vi "Logitech Camera.vi"() -> ()   [LabVIEW 2012]
uses:
  <vilib>/Utility/sysdir.llb/System Directory Type.ctl
panel:
  in  "error in":errorcluster
  out "error out":errorcluster
  out "Lines":T1(array[cluster]) {"End Point"."Y" format="%.2f"; "End Point"."X" format="%.2f"; "Start Point"."Y" format="%.2f"; "Start Point"."X" format="%.2f"}
  in  "stop?":bool caption="Stop (F)"
  out "Image Out":T2(plugin-control)
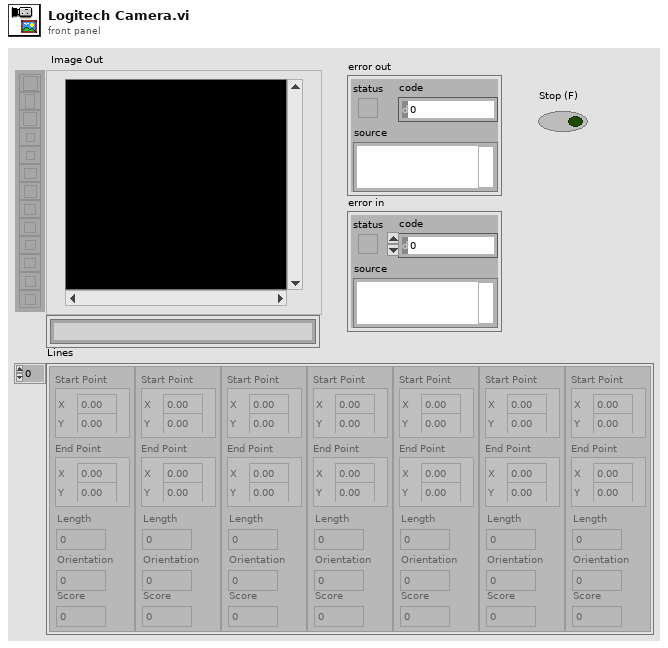
[diagram p1: front panel]
types:
  T1 = cluster{"Start Point":cluster{"X":sgl, "Y":sgl}, "End Point":cluster{"X":sgl, "Y":sgl}, "Length":dbl, "Orientation":dbl, "Score":dbl}[]
  T2 = typedef "IMAQ Image.ctl" = refnum<image>
  T3 = typedef "System Directory Type.ctl" = i32
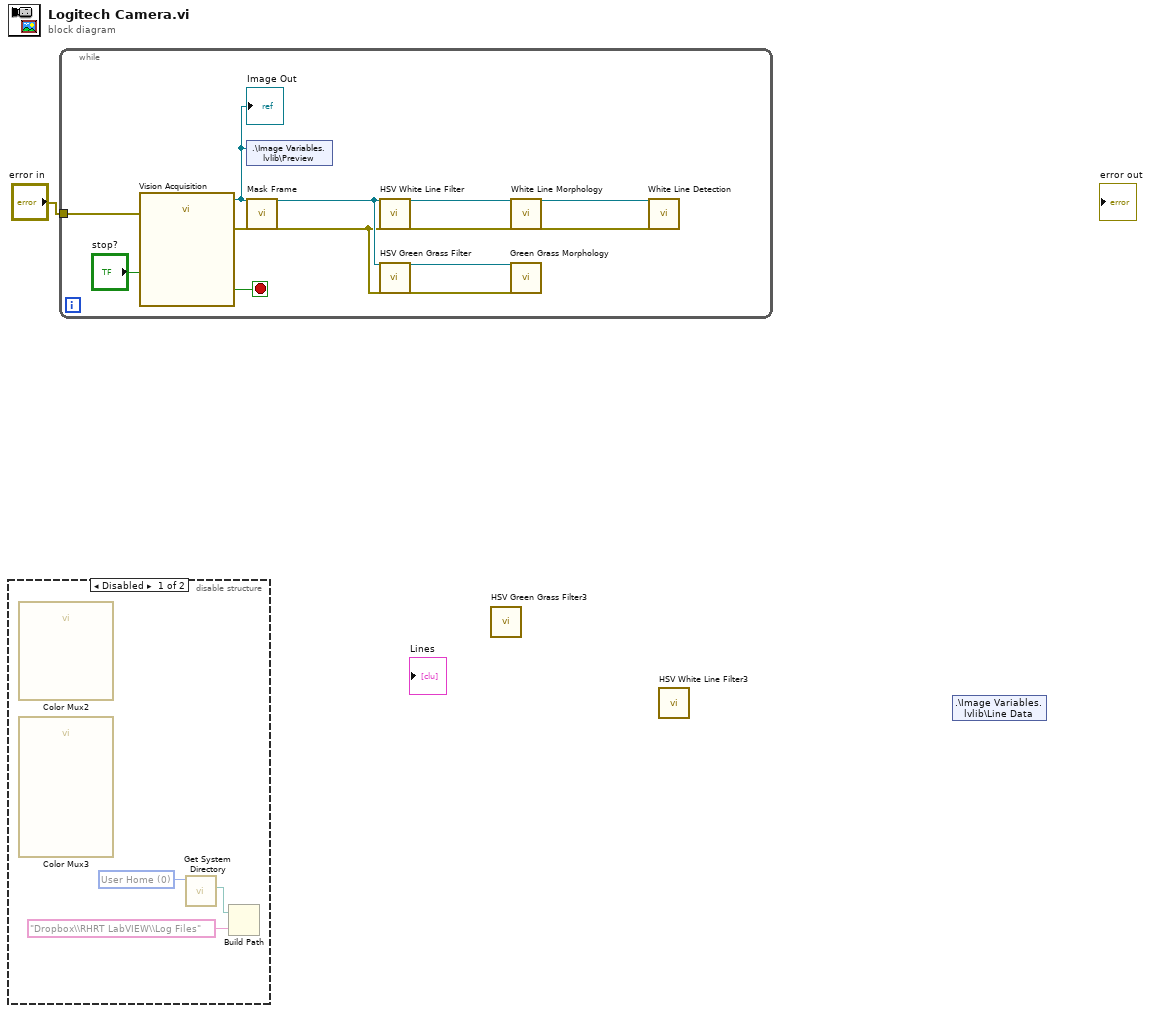
[diagram p0: block diagram]
diagram:
  n1 = disable-structure shown="Disabled" {
    frame Disabled {
      w2 = T3 0 items=["User Home"=0, "User Desktop"=1, "User Documents"=2, "User Application Data"=3, "User Preferences"=4, "User Temporary"=5, "Public Documents"=6, "Public Application Data"=7, "Public Preferences"=8, "Public Cache"=13, "System Core Libraries"=9, "System Installed Libraries"=10, "Application Files"=11, "Boot Volume Root"=12] ("system directory type")
      n2 = call "Color Mux2"() -> ()  [unwired: 26 in, 2 out]
      n3 = call "Color Mux3"() -> ()  [unwired: 23 in, 5 out]
      n4 = call <vilib>:"Get System Directory.vi"("system directory type"=w2) -> ("system directory"=w3:path)  [unwired: 10 in]
      n5 = Build Path(base path=w3, name or relative path="Dropbox\\RHRT LabVIEW\\Log Files") -> ()  [unwired: 1 out]
    }
    frame Enabled {
    }
  }
  n6 = while {
    tunnel: "error in" -> [w15]
    stop <- w16 stop-if-true
    n7 = call "Vision Acquisition"("Stop (F)"="stop?", "error in"=w15) -> ("Image Out"=w14:T2, "Stopped"=w16:bool, "error out"=w13:errorcluster)  [unwired: 23 in]
    "Image Out" <- w14
    n8 = shared-variable ".\\Image Variables.lvlib\\Preview"(w14) -> ()  [unwired: 1 in, 1 out]
    n9 = call "Mask Frame"("Image In"=w14, "error in"=w13) -> ("Image Out"=w8:T2, "error out"=w7:errorcluster)  [unwired: 24 in]
    n10 = call "HSV White Line Filter"("Image In"=w8, "error in"=w7) -> ("Image Out"=w12:T2, "error out"=w11:errorcluster)  [unwired: 24 in]
    n11 = call "HSV Green Grass Filter"("Image In"=w8, "error in"=w7) -> ("Image Out"=w6:T2, "error out"=w5:errorcluster)  [unwired: 24 in]
    n12 = call "White Line Morphology"("Image In"=w12, "error in"=w11) -> ("Image Out"=w10:T2, "error out"=w9:errorcluster)  [unwired: 24 in]
    n13 = call "Green Grass Morphology"("Image In"=w6, "error in"=w5) -> ()  [unwired: 24 in, 2 out]
    n14 = call "White Line Detection"("Image In"=w10, "error in"=w9) -> ()  [unwired: 22 in, 4 out]
  }
  n15 = call "HSV Green Grass Filter3"() -> ()  [unwired: 26 in, 2 out]
  n16 = call "HSV White Line Filter3"() -> ()  [unwired: 24 in, 4 out]
  n17 = shared-variable ".\\Image Variables.lvlib\\Line Data"() -> ()  [unwired: 2 in, 1 out]
